vi "Consumer.vi"(8 "error in (no error)":errorcluster, 9 "Data":variant, 10 "Case ID":string, 11 "uService Template in":refnum<class "Waiter.lvclass">) -> (0 "error out":errorcluster, 3 "uService Template out":refnum<class "Waiter.lvclass">)   [LabVIEW 2020, in "Waiter.lvlib" / "Waiter.lvclass"]
uses:
  Waiter.lvclass
  Waiter.lvclass/Waiter.ctl
  WaiterConsumer Case Selector.ctl
  TALOS/TALOS_PPL.lvlibp/Father of all uServices/Father of all uServices/Father of all uServices.lvclass
  TALOS/TALOS_PPL.lvlibp
  C:/LabVIEW Code/aegis-labview-code/TALOS/TALOS_PPL.lvlibp/Father of all uServices/Father of all uServices/Father of all uServices.lvclass
  C:/LabVIEW Code/aegis-labview-code/TALOS/TALOS_PPL.lvlibp/Ancestor/Ancestor/Ancestor.lvclass
  C:/LabVIEW Code/aegis-labview-code/TALOS/Actor Framework.lvlibp/1abvi3w/vi.lib/ActorFramework/Actor/Actor.lvclass
  C:/LabVIEW Code/aegis-labview-code/Other uServices/Waiter/Waiter.lvclass
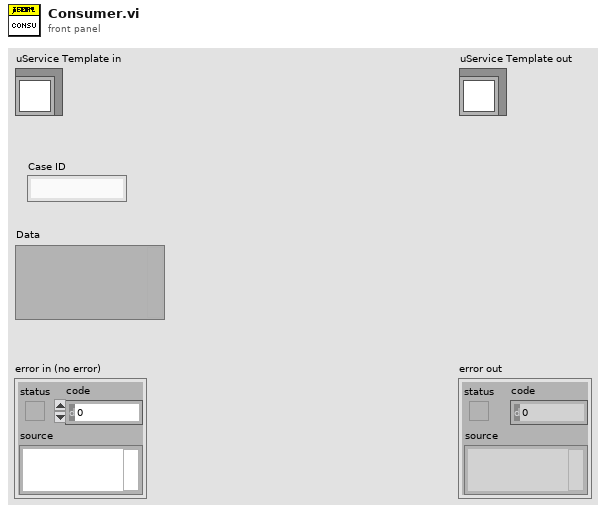
[diagram p1: front panel]
types:
  T1 = typedef "Waiter.lvlib/Waiter.lvclass/WaiterConsumer Case Selector.ctl" = enum16{"Send order to Pizza Machine"}
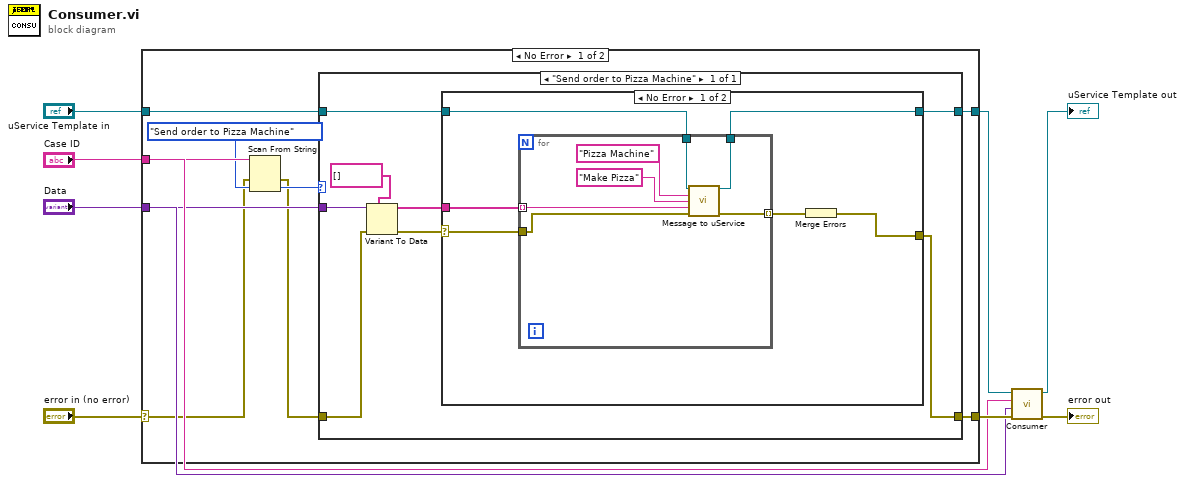
[diagram p0: block diagram]
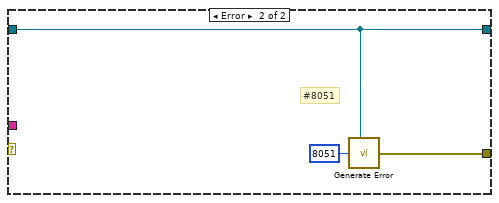
[diagram p2: hidden frame]
diagram:
  n1 = case shown="No Error" "error in (no error)" {
    selector: "error in (no error)" -> [w10 w42]
    tunnel: [w16 w43] -> w3
    tunnel: "uService Template in" -> [w17 w43]
    tunnel: [w14 w42] -> w6
    tunnel: "Case ID" -> [w13 _]
    tunnel: "Data" -> [w15 _]
    frame No Error {
      n2 = Scan From String(input string=w13, error in=w10, default 1=WaiterConsumer_Case_Selector."Send order to Pizza Machine" ("Consumer Case Selector")) -> (error out=w9:errorcluster, output 1=w11:T1)  [unwired: 2 in, 2 out]
      n3 = case shown="\"Send order to Pizza Machine\"" w11 {
        tunnel: w17 -> [w22]
        tunnel: [w19] -> w16
        tunnel: w15 -> [w25]
        tunnel: [w18] -> w14
        tunnel: w9 -> [w24]
        frame "Send order to Pizza Machine" {
          n4 = Variant To Data(error in=w24, type=string[] [], Variant=w25) -> (data=w20:string[], error out=w21:errorcluster)
          n5 = case shown="No Error" w21 {
            selector: w21 -> [w26 _]
            tunnel: w22 -> [w30 w39]
            tunnel: w20 -> [w31 _]
            tunnel: [w29 w39] -> w19
            tunnel: [w27 w40] -> w18
            frame No Error {
              n6 = for {
                tunnel: w31 -> [w34] mode=indexing
                tunnel: w30 -> [w38]
                tunnel: [w37] -> w29
                tunnel: [w33] -> w28 mode=indexing
                tunnel: w26 -> [w32]
                n7 = call "Message to uService.vi"("Father of all uServices in"=w38, "uService ID"="Pizza Machine", "Message"="Make Pizza", "Data"=w34, "error in (no error)"=w32) -> ("Father of all uServices out"=w37:refnum<class "Waiter.lvclass">, "error out"=w33:errorcluster)  [unwired: 9 in]
              }
              n8 = Merge Errors(w28) -> (w27:errorcluster)
            }
            frame Error {
              # "#8051"
              n9 = call "Generate Error.vi"("Class"=w39, "Error Code"=8051) -> ("error out"=w40:errorcluster)  [unwired: 5 in]
            }
          }
        }
      }
    }
    frame Error {
    }
  }
  n10 = call-parent "Consumer.vi"("error in (no error)"=w6, "Data"="Data", "Case ID"="Case ID", "uService Template in"=w3) -> ("error out"=→"error out":errorcluster, "uService Template out"=→"uService Template out":refnum<class "Waiter.lvclass">)  [unwired: 6 in]
